vi "Test2CalkiemDziala.vi"() -> ()   [LabVIEW 2020]
panel:
  out "Waveform Chart":dbl(graph)
  out "data out":string
  in  "stop":bool
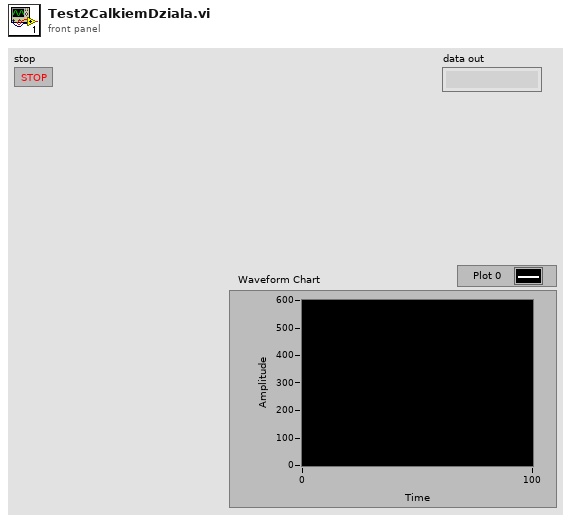
[diagram p1: front panel]
types:
  T1 = enum16{"Standard", "Buffered", "CRLF", "Immediate"}
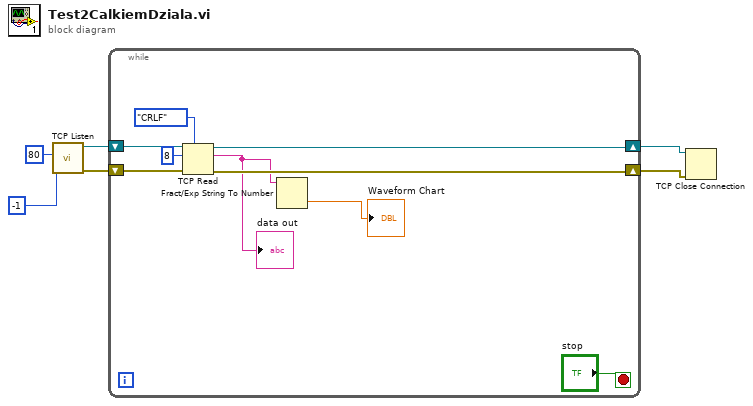
[diagram p0: block diagram]
diagram:
  n1 = call <vilib>:"TCP Listen.vi"("timeout ms (wait forever: -1)"=-1, "port"=u16 80) -> ("error out"=w5:errorcluster, "connection ID"=w6:refnum<k5>)  [unwired: 5 in, 3 out]
  n2 = while {
    shift-right: [w12] -> w3
    shift-left: w6 -> [w15]
    shift-right: [w13] -> w4
    shift-left: w5 -> [w14]
    stop <- "stop" stop-if-true
    n3 = TCP Read(connection ID=w15, bytes to read=8, error in (no error)=w14, 7:T1."CRLF" ("mode (standard)")) -> (connection ID out=w12:refnum<k5>, data out=w8:string, error out=w13:errorcluster)  [unwired: 1 in]
    "data out" <- w8
    n4 = Fract/Exp String To Number(string=w8) -> (number=→"Waveform Chart":dbl)  [unwired: 3 in, 1 out]
  }
  n5 = TCP Close Connection(connection ID=w3, error in (no error)=w4) -> ()  [unwired: 1 in, 2 out]
